vi "PCO_AllocateBuffer2.vi"(8 "error in (no error)":errorcluster, 9 "PointerSize (bytes)":u32=1447680, 10 "sBufNr":i16=-1, 11 "Handle":u64=136659496) -> (0 "error out":errorcluster, 1 "bytes allocated":u32, 2 "sBufNr out":i16, 3 "Handle Out":u64=136659496, 4 "BufferPointer":u64, 5 "return type":u32 format="%x")   [LabVIEW 2011]
uses:
  SC2_Cam64.dll
panel:
  # "A (hidden?) Labview function is used to allcoate the pointer"
  # "158334976"
  # "161284096"
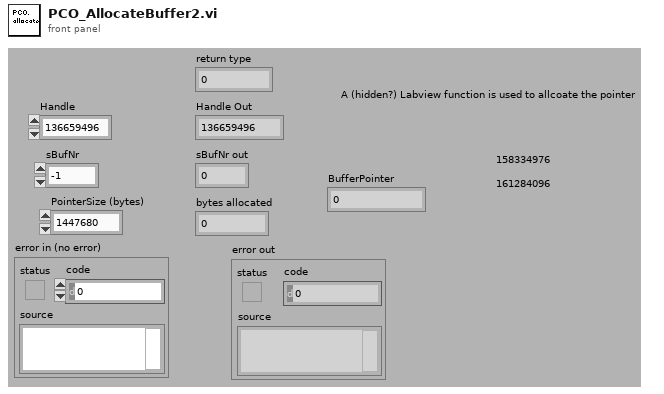
[diagram p1: front panel]
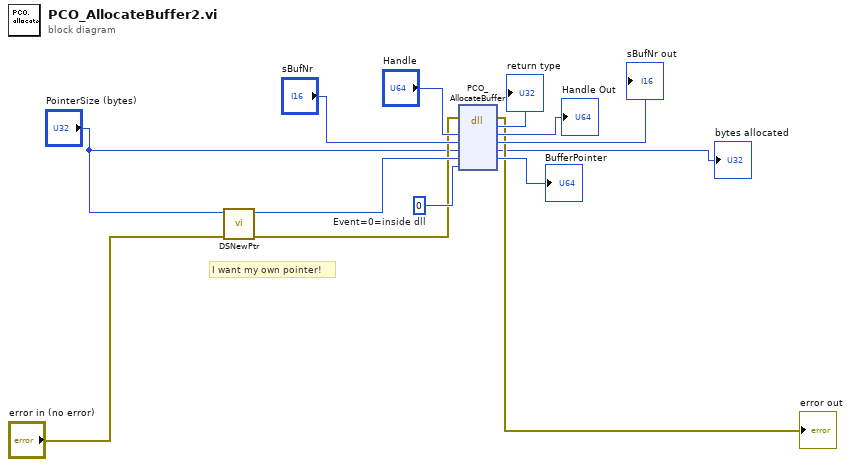
[diagram p0: block diagram]
diagram:
  w10 = 0  # Event=0=inside dll
  # "I want my own pointer!"
  n1 = call <vilib>:"DSNewPtr.vi"("error in (no error)"="error in (no error)", "Size"="PointerSize (bytes)") -> ("error out"=w3:errorcluster, "Pointer"=w5:u64)  [unwired: 8 in]
  n2 = dll-call lib="C:/Program Files/colibri/Drivers/PCO.Camera/SC2_Cam*.*" fn="PCO_AllocateBuffer"(error in=w3, "Handle"="Handle", "sBufNr"="sBufNr", "dwSize"="PointerSize (bytes)", "wBuf"=w5, "hEvent"=w10) -> (error out=→"error out":errorcluster, "return type"=→"return type":u32, "Handle"=→"Handle Out":u64, "sBufNr"=→"sBufNr out":i16, "dwSize"=→"bytes allocated":u32, "wBuf"=→"BufferPointer":u64)  [unwired: 2 in, 2 out]
